vi "CTRE_Phoenix_MotorControl_SetIntegratedSensorPosition_TalonFX_Polymorphic.vi"   [LabVIEW 2019]
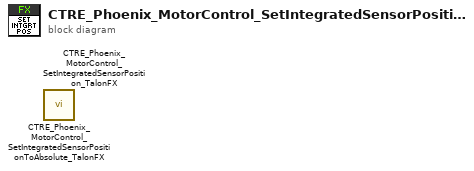
[diagram p0: block diagram]
diagram:
  n1 = call <vilib>:"CTRE_Phoenix_MotorControl_SetIntegratedSensorPositionToAbsolute_TalonFX.vi"() -> ()  [unwired: 10 in, 2 out]
  n2 = call <vilib>:"CTRE_Phoenix_MotorControl_SetIntegratedSensorPosition_TalonFX.vi"() -> ()  [unwired: 10 in, 2 out]
